vi "Parse XML Metadata From Cluster Record.vi"(5 "Node Reference":refnum<k20>) -> (0 "XML Data":string, 1 "Name":string, 2 "Version":string)   [LabVIEW 2013]
uses:
  <resource>/objmgr/DOMUserDefRef.rc
  <vilib>/xml/NI_XML.lvlib
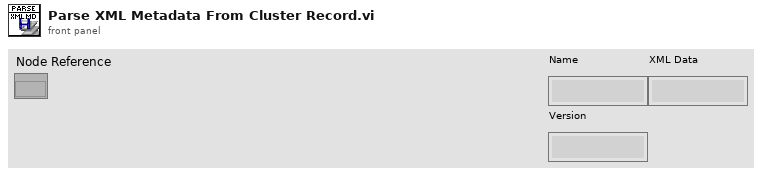
[diagram p1: front panel]
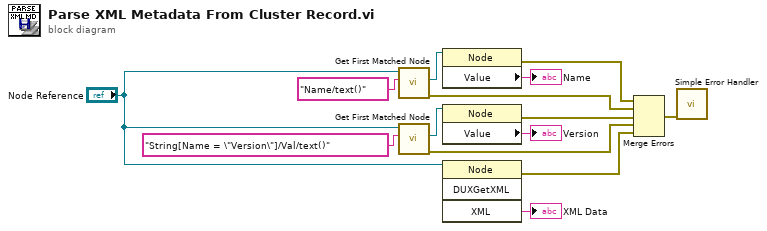
[diagram p0: block diagram]
diagram:
  n1 = call <vilib>:"Get First Matched Node.vi"("XPath expression"="Name/text()", "node in"="Node Reference") -> ("error out"=w5:errorcluster, "node result"=w12:refnum<k20>)  [unwired: 7 in, 1 out]
  n2 = call <vilib>:"Get First Matched Node.vi"("XPath expression"="String[Name = \"Version\"]/Val/text()", "node in"="Node Reference") -> ("error out"=w3:errorcluster, "node result"=w13:refnum<k20>)  [unwired: 7 in, 1 out]
  n3 = property class="Node"(reference=w12) -> (error out=w6:errorcluster, "Value"=→"Name":string)  [unwired: 1 in, 1 out]
  n4 = property class="Node"(reference=w13) -> (error out=w4:errorcluster, "Value"=→"Version":string)  [unwired: 1 in, 1 out]
  n5 = invoke class="Node" method="DUXGetXML"(reference="Node Reference") -> (error out=w2:errorcluster, "XML"=→"XML Data":string)  [unwired: 3 in, 2 out]
  n6 = Merge Errors(w6, w5, w4, w3, w2) -> (w1:errorcluster)
  n7 = call <vilib>:"Simple Error Handler.vi"("error in (no error)"=w1) -> ()  [unwired: 4 in, 5 out]
